vi "sub_DTMF_StringToNumber.vi"(11 "Phone # String":string) -> (3 "Phone Number":u8[](array[numeric]))   [LabVIEW 2011]
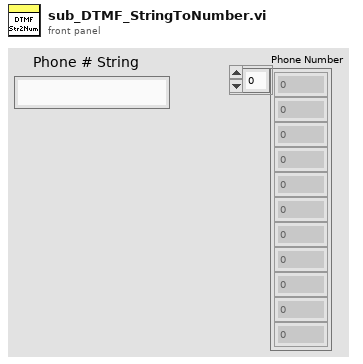
[diagram p1: front panel]
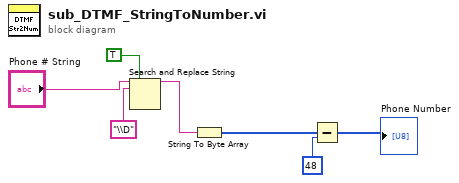
[diagram p0: block diagram]
diagram:
  n1 = Search and Replace String(replace all?=TRUE ("replace all? (F)"), input string="Phone # String", search string="\\D") -> (result string=w5:string)  [unwired: 5 in, 3 out]
  n2 = String To Byte Array(string=w5) -> (unsigned byte array=w3:u8[])
  n3 = Subtract(x=w3, y=48) -> (x-y=→"Phone Number":i32[])
